vi "Pos01.vi"(7 "Version":string, 9 "Local Origin":cluster{"X":dbl, "Y":dbl, "Z":dbl}, 11 "String":string) -> (1 "W-Pos":cluster{"X":dbl, "Y":dbl, "Z":dbl}, 2 "M-Pos":cluster{"X":dbl, "Y":dbl, "Z":dbl})   [LabVIEW 2019]
panel:
  out "remaining string":string
  out "after substring":string
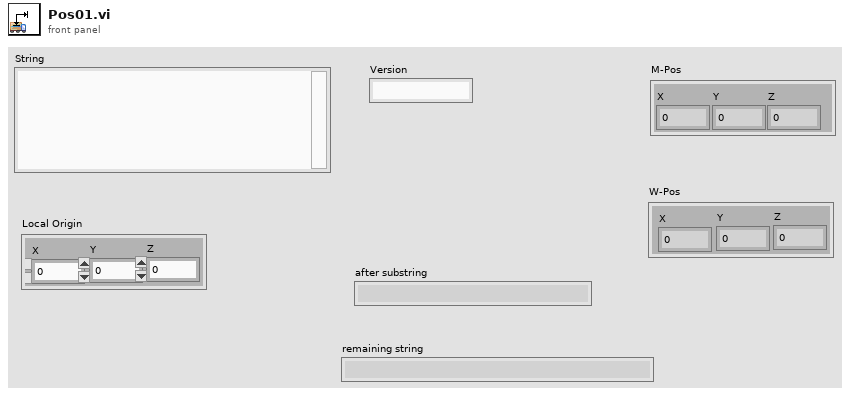
[diagram p1: front panel]
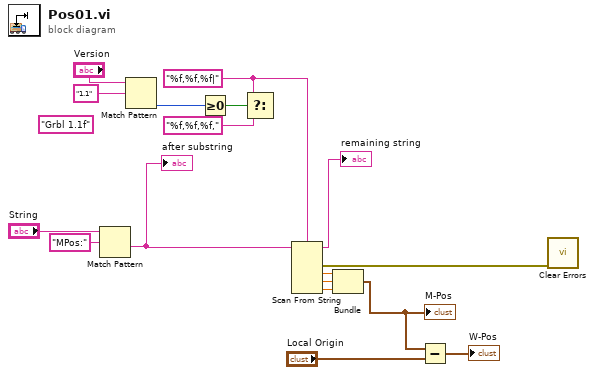
[diagram p0: block diagram]
diagram:
  (unwired) "Grbl 1.1f" ("Version")
  w6 = "%f,%f,%f|" ("format string")
  n1 = Match Pattern(string="String", regular expression="MPos:") -> (after substring=w16:string)  [unwired: 1 in, 3 out]
  "after substring" <- w16
  n2 = Match Pattern(string="Version", regular expression="1.1" ("Version")) -> (offset past match=w2:i32)  [unwired: 1 in, 3 out]
  n3 = Greater Or Equal To 0?(x=w2) -> (x >= 0?=w1:bool)
  n4 = Select(t=w6, s=w1, f="%f,%f,%f," ("format string")) -> ()  [unwired: 1 out]
  n5 = Scan From String(format string=w6, input string=w16) -> (remaining string=→"remaining string":string, error out=w10:errorcluster, output 1=w13:dbl, output 2=w11:dbl, output 3=w12:dbl)  [unwired: 5 in, 1 out]
  n6 = Bundle(w13, w11, w12) -> (w9:cluster{dbl, dbl, dbl})  [unwired: 1 in]
  "M-Pos" <- w9
  n7 = Subtract(x=w9, y="Local Origin") -> (x-y=→"W-Pos":cluster{dbl, dbl, dbl})
  n8 = call <vilib>:"Clear Errors.vi"("error in (no error)"=w10) -> ()  [unwired: 5 in, 2 out]
